vi "Kinect Code.vi"() -> ()   [LabVIEW 2014]
uses:
  Wrapper/Wrapper/CreateContext.vi
  Wrapper/Wrapper/Initialise Depth.vi
  Wrapper/Wrapper/GetDepth.vi
panel:
  in  "STOP":errorcluster
  out "error out":errorcluster
  out "FrameID":i32
  out "Depth":i32(graph)
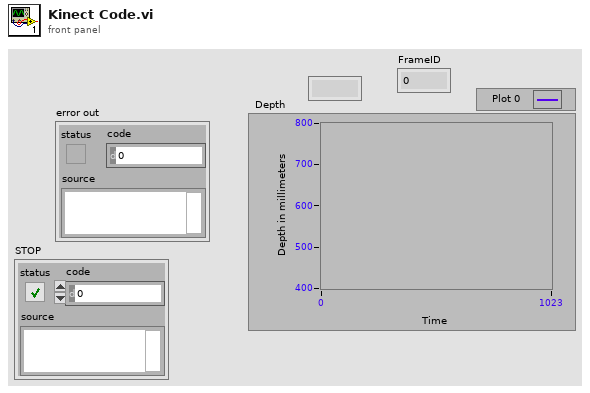
[diagram p1: front panel]
types:
  T1 = enum16{"big-endian, network order", "native, host order", "little-endian"}
  T2 = typedef "Control Kinect Refs.ctl" = cluster{"Context":refnum<k24>, "DepthGenerator":refnum<k24>, "DepthMetaData":refnum<k24>, "MapOutputMode":refnum<k24>, "ImageGenerator":refnum<k24>, "ImageMetaData":refnum<k24>, "UserGenerator":refnum<k24>, "SkeletonCapability":refnum<k24>, "PoseDetectionCapability":refnum<k24>, "SkeletonJoint":refnum<k24>, "SkeletonJointPosition":refnum<k24>, "Point3D":refnum<k24>, "NewUser event":refnum<k27>, "PoseDetected event":refnum<k27>, "CalibrationEnd event":refnum<k27>}
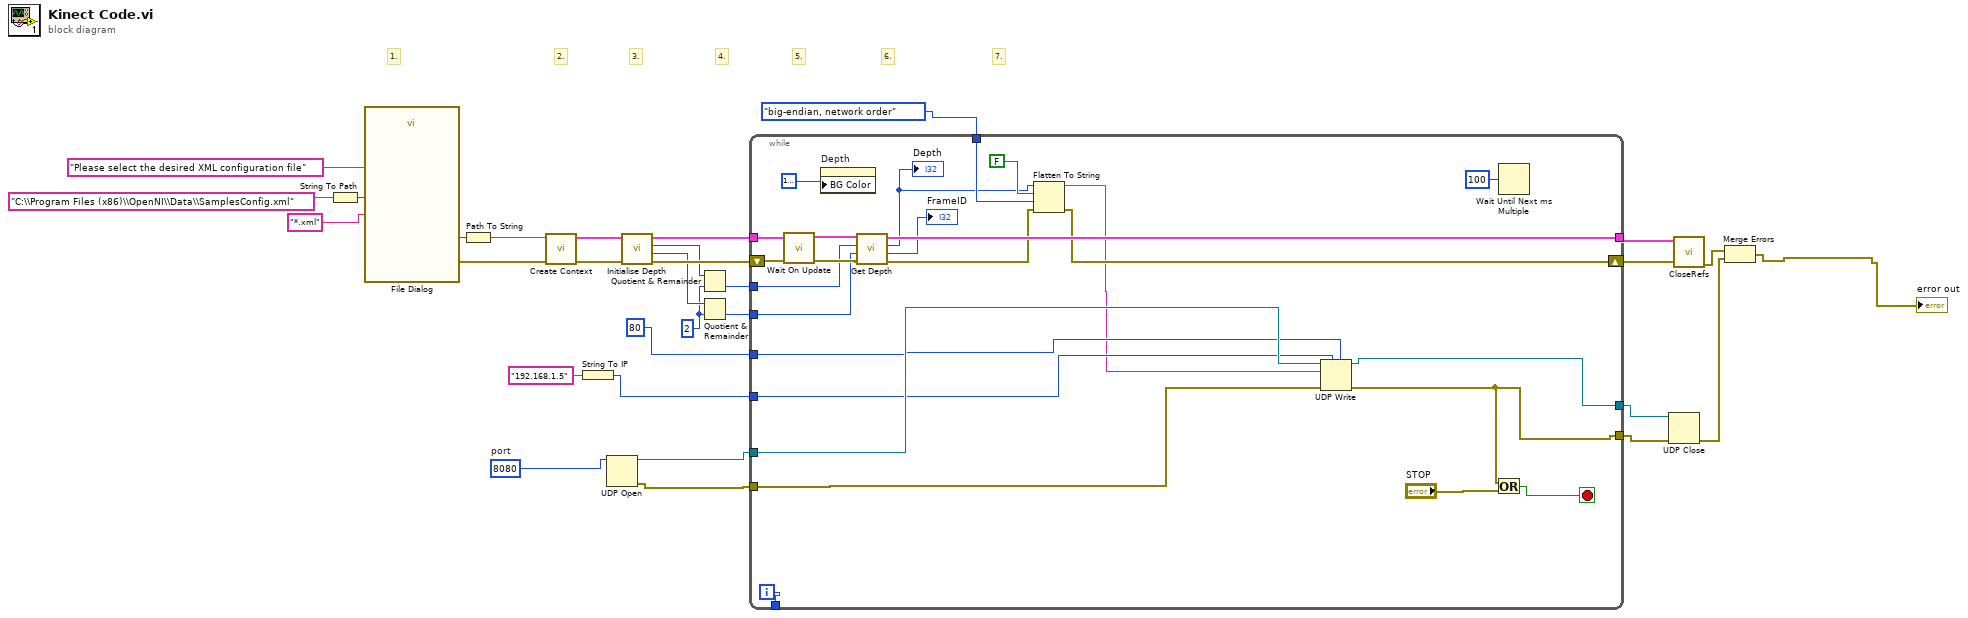
[diagram p0: block diagram]
diagram:
  w1 = u16 8080  # port
  w16 = 2
  # "5."
  # "6."
  # "7."
  # "4."
  # "3."
  # "2."
  # "1."
  n1 = String To Path(string="C:\\Program Files (x86)\\OpenNI\\Data\\SamplesConfig.xml") -> (path=w29:path)
  n2 = call "File Dialog"("start path"=w29, "prompt"="Please select the desired XML configuration file", "pattern (all files)"="*.xml") -> ("selected path"=w26:path, "error out"=w24:errorcluster)  [unwired: 9 in, 2 out]
  n3 = Path To String(path=w26) -> (string=w25:string)
  n4 = call "Create Context"("error in"=w24, "Path to configuration"=w25) -> ("error out"=w21:errorcluster, "Kinect References out"=w22:T2)  [unwired: 8 in]
  n5 = String To IP(1:"192.168.1.5" ("name")) -> (0:w2:u32)
  n6 = UDP Open(11:w1) -> (port=w4:refnum<k16>, 0:w5:errorcluster)  [unwired: 4 in, 1 out]
  n7 = call "Initialise Depth"("error in (no error)"=w21, "Kinect References in"=w22) -> ("error out"=w19:errorcluster, "YRes"=w17:i32, "XRes"=w18:i32, "Kinect References out"=w20:T2)  [unwired: 6 in]
  n8 = Quotient & Remainder(x=w18, y=w16) -> (floor(x/y)=w15:i32)  [unwired: 1 out]
  n9 = Quotient & Remainder(x=w17, y=w16) -> (floor(x/y)=w14:i32)  [unwired: 1 out]
  n10 = while {
    tunnel: w20 -> [w53]
    tunnel: [w55] -> w13
    shift-right: [w45] -> w12
    shift-left: w19 -> [w44]
    tunnel: w15 -> [w49]
    tunnel: w14 -> [w50]
    tunnel: T1."big-endian, network order" ("byte order (0:big-endian, network order)") -> [w36]
    tunnel: [w41] -> w9
    tunnel: [w39] -> w10
    tunnel: [w43] -> _
    tunnel: w4 -> [w42]
    tunnel: w2 -> [w34]
    tunnel: w5 -> [w37]
    tunnel: u32 80 -> [w35]
    i -> [w43]
    stop <- w40 stop-if-true
    n11 = call "Wait On Update.vi"("error in"=w44, "Kinect References in"=w53) -> ("error out"=w51:errorcluster, "Kinect References out"=w52:T2)  [unwired: 8 in]
    n12 = property on="Depth" class="WFChart (strict)"("BG Color"=u32 16777216) -> ()  [unwired: 2 in, 2 out]
    n13 = call "Get Depth"("error in (no error)"=w51, "Y"=w50, "X"=w49, "Kinect References in"=w52) -> ("error out"=w46:errorcluster, "FrameID"=→"FrameID":i32, "Depth"=w33:i32, "Kinect References out"=w55:T2)  [unwired: 4 in]
    "Depth" <- w33
    n14 = Flatten To String(anything=w33, prepend array or string size? (T)=FALSE, byte order (0:big-endian, network order)=w36, error in (no error)=w46) -> (data string=w32:string, error out=w45:errorcluster)  [unwired: 1 out]
    n15 = UDP Write(address=w34, port or service name=w35, connection ID=w42, data in=w32, 8:w37) -> (error out=w39:errorcluster, 3:w41:refnum<k16>)  [unwired: 1 in]
    n16 = Or(x=w39, y="STOP") -> (x .or. y?=w40:bool)
    n17 = Wait Until Next ms Multiple(millisecond multiple=u32 100) -> ()  [unwired: 1 out]
  }
  n18 = UDP Close(connection ID=w9, 8:w10) -> (error out=w7:errorcluster)  [unwired: 1 out]
  n19 = call "CloseRefs.vi"("error in (no error)"=w12, "Kinect References in"=w13) -> ("error out"=w8:errorcluster)  [unwired: 9 in]
  n20 = Merge Errors(w8, w7) -> (→"error out":errorcluster)
